vi "Read Config File.vi"(8 "error in (no error)":errorcluster) -> (0 "error out":errorcluster, 1 "Config File Sort":string, 2 "Legend out":cluster{"Color Box":u32, "String":string}[](array[cluster]), 3 "Data Folder Path":path)   [LabVIEW 2018]
uses:
  <vilib>/Utility/config.llb/Write Key (String).vi
  <vilib>/Utility/config.llb/Write Key (Path).vi
  <vilib>/Utility/config.llb/Write Key (U32).vi
  <vilib>/Utility/config.llb/Read Key (Path).vi
  <vilib>/Utility/config.llb/Read Key (String).vi
  <vilib>/Utility/config.llb/Read Key (U32).vi
  <vilib>/Utility/config.llb/NI_LVConfig.lvlib
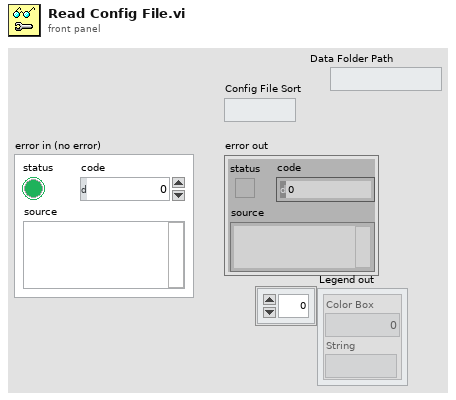
[diagram p1: front panel]
types:
  T1 = typedef "NI_LVConfig.lvlib/Config Data RefNum.ctl" = refnum<k1>
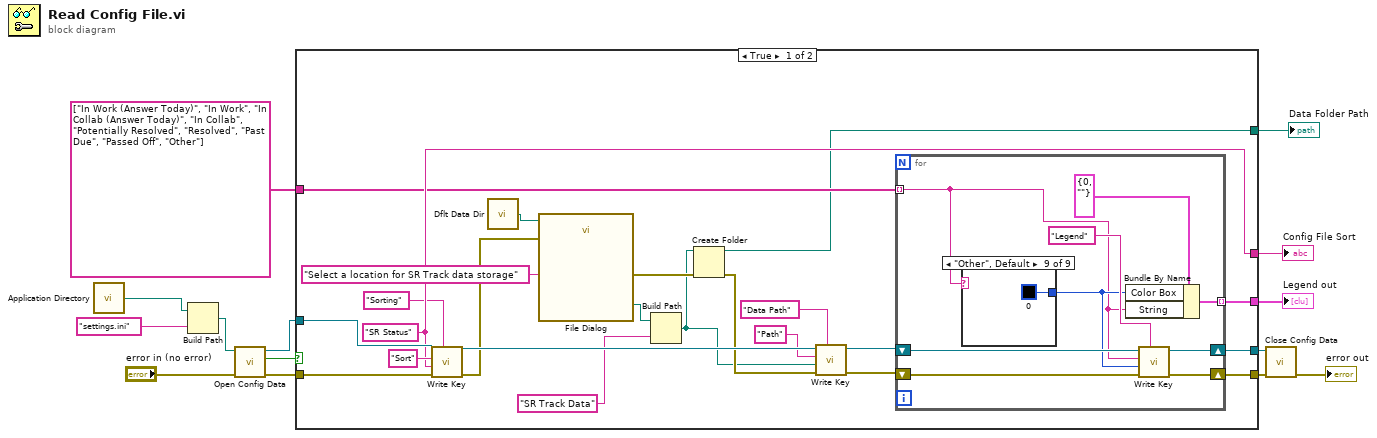
[diagram p0: block diagram]
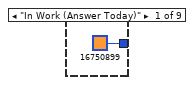
[diagram p2: hidden frame]
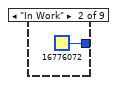
[diagram p3: hidden frame]
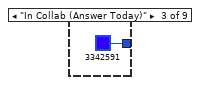
[diagram p4: hidden frame]
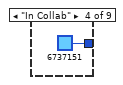
[diagram p5: hidden frame]
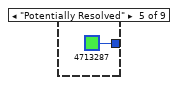
[diagram p6: hidden frame]
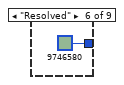
[diagram p7: hidden frame]
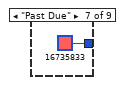
[diagram p8: hidden frame]
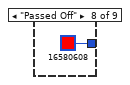
[diagram p9: hidden frame]
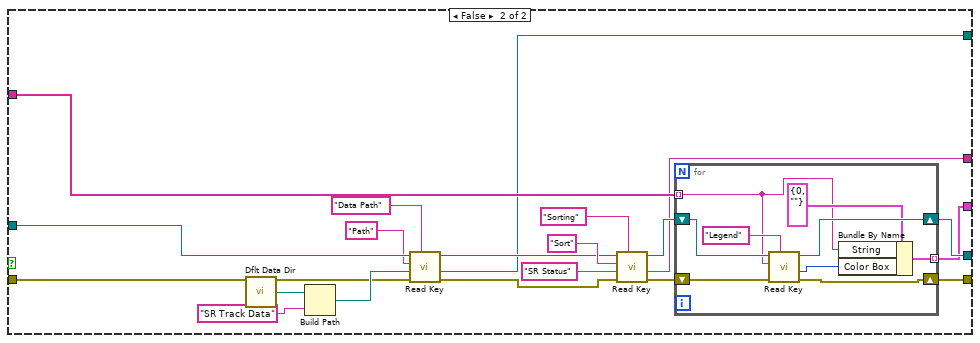
[diagram p10: hidden frame]
diagram:
  n1 = call <vilib>:"Application Directory.vi"() -> ("Application Directory"=w4:path)
  n2 = Build Path(base path=w4, name or relative path="settings.ini") -> (appended path=w6:path)
  n3 = call <vilib>:"Open Config Data.vi"("error in (no error)"="error in (no error)", "configuration file path"=w6) -> ("error out"=w8:errorcluster, "file created?"=w7:bool, "refnum"=w1:T1)  [unwired: 7 in]
  n4 = case shown="True" w7 {
    tunnel: w1 -> [w37 w64]
    tunnel: w8 -> [w35 w59]
    tunnel: [w34 w68] -> w9
    tunnel: [w33 w73] -> w10
    tunnel: [w32 w71] -> w11
    tunnel: string[] ["In Work (Answer Today)", "In Work", "In Collab (Answer Today)", "In Collab", "Potentially Resolved", "Resolved", "Past Due", "Passed Off", "Other"] -> [w31 w70]
    tunnel: [w30 w67] -> w3
    tunnel: [w18 w63] -> w2
    frame True {
      w34 = "SR Status" ("key")
      n5 = call-poly <vilib>:"Write Key.vi"("section"="Sorting", "error in (no error)"=w35, "value"=w34, "key"="Sort", "refnum"=w37) -> ("error out"=w22:errorcluster, "refnum out"=w26:T1)  [unwired: 4 in, 1 out]
      n6 = call <vilib>:"Dflt Data Dir.vi"() -> ("App:Default Data Directory"=w23:path)
      n7 = call "File Dialog"("start path"=w23, "prompt"="Select a location for SR Track data storage", "error in"=w22) -> ("selected path"=w17:path, "error out"=w16:errorcluster)  [unwired: 9 in, 2 out]
      n8 = Build Path(base path=w17, name or relative path="SR Track Data" ("prompt")) -> (appended path=w15:path)
      n9 = Create Folder(path (use dialog)=w15, error in=w16) -> (created path=w18:path, error out=w19:errorcluster)  [unwired: 1 in, 1 out]
      n10 = call-poly <vilib>:"Write Key.vi"("section"="Data Path", "error in (no error)"=w19, "value"=w15, "key"="Path", "refnum"=w26) -> ("error out"=w27:errorcluster, "refnum out"=w28:T1)  [unwired: 4 in, 1 out]
      n11 = for {
        shift-right: [w46] -> w33
        shift-left: w28 -> [w44]
        shift-right: [w42] -> w32
        shift-left: w27 -> [w43]
        tunnel: w31 -> [w39] mode=indexing
        tunnel: [w38] -> w30 mode=indexing
        n12 = case shown="\"Other\", Default" w39 {
          tunnel: [u32 16750899 u32 16776072 u32 3342591 u32 6737151 u32 4713287 u32 9746580 u32 16735833 u32 16580608 u32 0] -> w40
          frame "In Work (Answer Today)" {
          }
          frame "In Work" {
          }
          frame "In Collab (Answer Today)" {
          }
          frame "In Collab" {
          }
          frame "Potentially Resolved" {
          }
          frame "Resolved" {
          }
          frame "Past Due" {
          }
          frame "Passed Off" {
          }
          frame "Other", Default {
          }
        }
        n13 = Bundle By Name(cluster=cluster{"Color Box":u32, "String":string} {"Color Box"=0, "String"=""} ("element"), "Color Box"=w40, "String"=w39) -> (w38:cluster{"Color Box":u32, "String":string})
        n14 = call-poly <vilib>:"Write Key.vi"("section"="Legend", "error in (no error)"=w43, "value"=w40, "key"=w39, "refnum"=w44) -> ("error out"=w42:errorcluster, "refnum out"=w46:T1)  [unwired: 4 in, 1 out]
      }
    }
    frame False {
      n15 = call <vilib>:"Dflt Data Dir.vi"() -> ("App:Default Data Directory"=w56:path)
      n16 = Build Path(base path=w56, name or relative path="SR Track Data" ("prompt")) -> (appended path=w60:path)
      n17 = call-poly <vilib>:"Read Key.vi"("section"="Data Path", "error in (no error)"=w59, "default value"=w60, "key"="Path", "refnum"=w64) -> ("error out"=w58:errorcluster, "value"=w63:path, "refnum out"=w65:T1)  [unwired: 3 in, 1 out]
      n18 = call-poly <vilib>:"Read Key.vi"("section"="Sorting", "error in (no error)"=w58, "default value"="SR Status" ("key"), "key"="Sort", "refnum"=w65) -> ("error out"=w72:errorcluster, "value"=w68:string, "refnum out"=w74:T1)  [unwired: 3 in, 1 out]
      n19 = for {
        shift-right: [w84] -> w73
        shift-left: w74 -> [w82]
        shift-right: [w80] -> w71
        shift-left: w72 -> [w81]
        tunnel: w70 -> [w77] mode=indexing
        tunnel: [w78] -> w67 mode=indexing
        n20 = call-poly <vilib>:"Read Key.vi"("section"="Legend", "error in (no error)"=w81, "key"=w77, "refnum"=w82) -> ("error out"=w80:errorcluster, "value"=w76:u32, "refnum out"=w84:T1)  [unwired: 4 in, 1 out]
        n21 = Bundle By Name(cluster=cluster{"Color Box":u32, "String":string} {"Color Box"=0, "String"=""} ("element"), "String"=w77, "Color Box"=w76) -> (w78:cluster{"Color Box":u32, "String":string})
      }
    }
  }
  "Config File Sort" <- w9
  "Legend out" <- w3
  "Data Folder Path" <- w2
  n22 = call <vilib>:"Close Config Data.vi"("error in (no error)"=w11, "refnum"=w10) -> ("error out"=→"error out":errorcluster)  [unwired: 8 in, 1 out]
